vi "Initialize.vi"(7 "Simulate?":bool, 8 "error in (no error)":errorcluster, 10 "Port config":T1={"baud rate"=9600, "data bits"=8, "parity"=enum."None", "stop bits"=0}, 11 "VISA Refnum in":refnum<visa-resource-name>) -> (0 "error out":errorcluster, 2 "Connected?":bool, 3 "VISA Refnum out":refnum<visa-resource-name>)   [LabVIEW 2020, in "Monochromator.lvlib"]
uses:
  Monochromator.lvlib
  <vilib>/Instr/_visa.llb/VISA Flush IO Buffer Mask.ctl
  <vilib>/Instr/_visa.llb/VISA Configure Serial Port (Instr).vi
panel:
  out "return count write":u32
  out "return count read":u32
  out "Data read":string
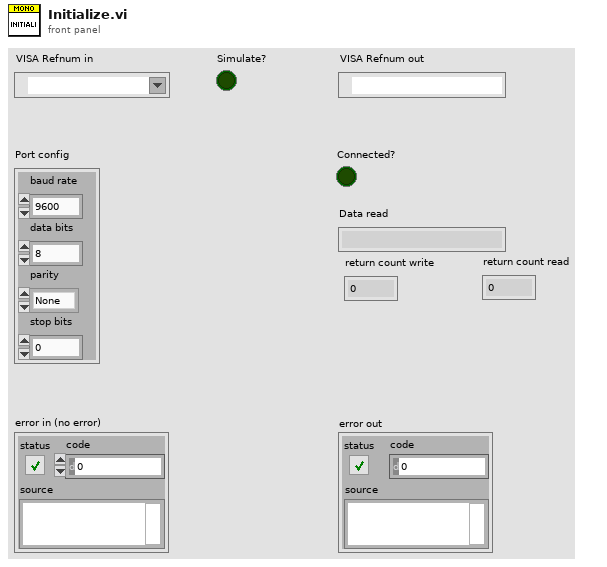
[diagram p1: front panel]
types:
  T1 = cluster{"baud rate":u32, "data bits":u16, "parity":enum16{"None", "Odd", "Even", "Mark", "Space"}, "stop bits":u16}
  T2 = typedef "VISA Flush IO Buffer Mask.ctl" = u16
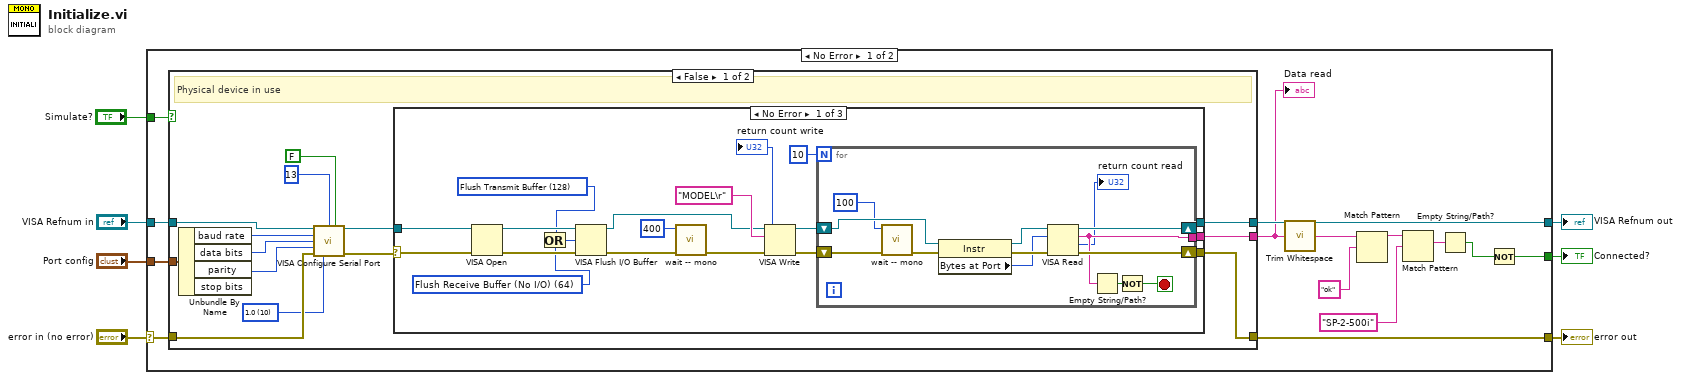
[diagram p0: block diagram]
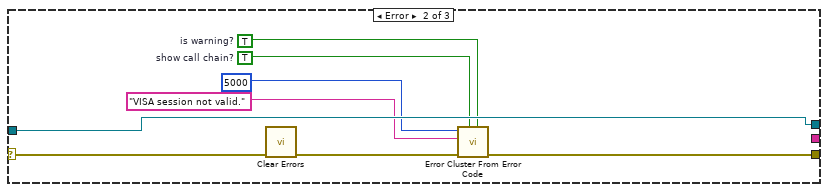
[diagram p2: hidden frame]
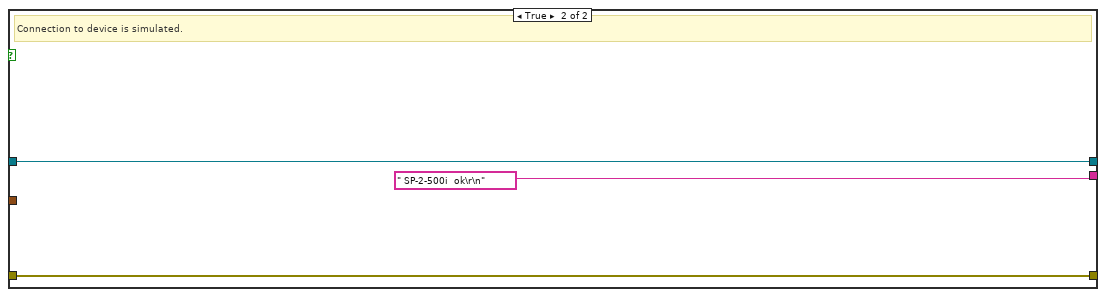
[diagram p4: hidden frame]
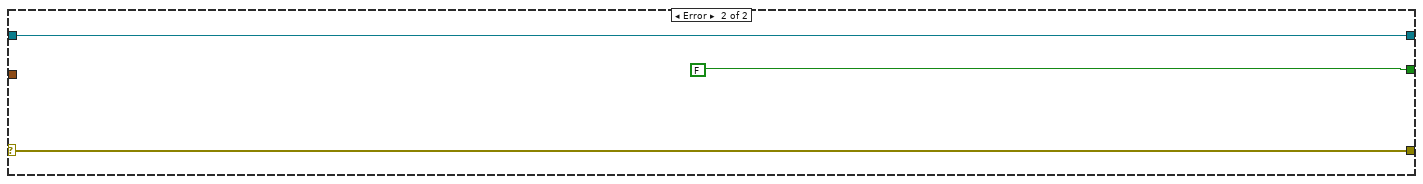
[diagram p5: hidden frame]
diagram:
  n1 = case shown="No Error" "error in (no error)" {
    selector: "error in (no error)" -> [w19 w82]
    tunnel: "Port config" -> [w21 _]
    tunnel: "VISA Refnum in" -> [w20 w83]
    tunnel: [w18 w82] -> w4
    tunnel: [w17 w83] -> w3
    tunnel: [w9 FALSE] -> w2
    tunnel: "Simulate?" -> [w8 _]
    frame No Error {
      n2 = case shown="False" w8 {
        tunnel: w21 -> [w35 _]
        tunnel: w20 -> [w34 w78]
        tunnel: w19 -> [w33 w79]
        tunnel: [w32 w79] -> w18
        tunnel: [w31 w78] -> w17
        tunnel: [w30 " SP-2-500i  ok\r\n" ("regular expression")] -> w15
        frame False {
          w25 = u16 10 items=["1.0"=10, "1.5"=15, "2.0"=20] ("stop bits (10: 1 bit)")
          # "Physical device in use"
          n3 = Unbundle By Name(w35) -> ("baud rate"=w27:u32, "data bits"=w28:u16, "parity"=w29:enum16{"None", "Odd", "Even", "Mark", "Space"})  [unwired: 1 out]
          n4 = call-poly "VISA Configure Serial Port"("VISA resource name"=w34, "termination char\n(0xA = '\\n' = LF)"=u8 13 ("termination char\n(0xA = '\\n' = LF)"), "Enable Termination\nChar (T)"=FALSE ("Enable Termination\nChar (T)"), "baud rate (9600)"=w27, "data bits (8)"=w28, "parity (0:none)"=w29, "error in (no error)"=w33, "stop bits (10: 1 bit)"=w25) -> ("VISA resource name out"=w24:refnum<visa-resource-name>, "error out"=w23:errorcluster)  [unwired: 6 in]
          n5 = case shown="No Error" w23 {
            selector: w23 -> [w50 w74 w76]
            tunnel: [w54 w72 w76] -> w32
            tunnel: [w53 w75 w77] -> w31
            tunnel: [w52 _ _] -> w30
            tunnel: w24 -> [w51 w75 w77]
            frame No Error {
              w38 = T2 64 items=["Flush Receive Buffer"=16, "Write Transmit Buffer to Device"=32, "Flush Receive Buffer (No I/O)"=64, "Flush Transmit Buffer"=128] ("Mask")
              w39 = T2 128 items=["Flush Receive Buffer"=16, "Write Transmit Buffer to Device"=32, "Flush Receive Buffer (No I/O)"=64, "Flush Transmit Buffer"=128] ("Mask")
              n6 = VISA Open(error in (no error)=w50, VISA resource name=w51) -> (VISA resource name=w41:refnum<visa-resource-name>, error out=w43:errorcluster)  [unwired: 3 in]
              n7 = Or(x=w39, y=w38) -> (x .or. y?=w37:T2)
              n8 = VISA Flush I/O Buffer(VISA resource name=w41, mask (16)=w37, error in (no error)=w43) -> (VISA resource name out=w40:refnum<visa-resource-name>, error out=w42:errorcluster)
              n9 = call "wait -- mono.vi"("error in (no error)"=w42, "milliseconds to wait"=u32 400) -> ("error out"=w46:errorcluster)  [unwired: 9 in]
              n10 = VISA Write(VISA resource name=w40, write buffer="MODEL\r", error in (no error)=w46) -> (VISA resource name out=w49:refnum<visa-resource-name>, return count=→"return count write":u32, error out=w48:errorcluster)
              n11 = for {
                N: 10 -> [_]
                tunnel: [w58] -> w52
                shift-right: [w66] -> w53
                shift-left: w49 -> [w64]
                shift-right: [w67] -> w54
                shift-left: w48 -> [w62]
                stop <- w56 stop-if-true
                n12 = call "wait -- mono.vi"("error in (no error)"=w62, "milliseconds to wait"=u32 100) -> ("error out"=w61:errorcluster)  [unwired: 9 in]
                n13 = property class="Instr"(reference=w64, error in=w61) -> (reference out=w63:refnum<visa-resource-name>, error out=w65:errorcluster, "Bytes at Port"=w59:u32)
                n14 = VISA Read(VISA resource name=w63, byte count=w59, error in (no error)=w65) -> (VISA resource name out=w66:refnum<visa-resource-name>, read buffer=w58:string, return count=→"return count read":u32, error out=w67:errorcluster)
                n15 = Empty String/Path?(string/path=w58) -> (empty?=w57:bool)
                n16 = Not(x=w57) -> (.not. x?=w56:bool)
              }
            }
            frame Error {
              w68 = TRUE  # show call chain?
              w69 = TRUE  # is warning?
              n17 = call <vilib>:"Clear Errors.vi"("error in (no error)"=w74) -> ("error out"=w73:errorcluster)  [unwired: 5 in, 1 out]
              n18 = call <vilib>:"Error Cluster From Error Code.vi"("is warning? (False)"=w69, "show call chain? (False)"=w68, "error in (no error)"=w73, "error message (\"\")"="VISA session not valid." ("error message (\"\")"), "error code (0)"=5000) -> ("error out"=w72:errorcluster)  [unwired: 4 in]
            }
            frame Default {
            }
          }
        }
        frame True {
          # "Connection to device is simulated."
        }
      }
      "Data read" <- w15
      n19 = call <vilib>:"Trim Whitespace.vi"("string"=w15) -> ("trimmed string"=w14:string)  [unwired: 1 in]
      n20 = Match Pattern(string=w14, regular expression="ok") -> (before substring=w13:string)  [unwired: 1 in, 3 out]
      n21 = Match Pattern(string=w13, regular expression="SP-2-500i" ("y")) -> (match substring=w11:string)  [unwired: 1 in, 3 out]
      n22 = Empty String/Path?(string/path=w11) -> (empty?=w10:bool)
      n23 = Not(x=w10) -> (.not. x?=w9:bool)
    }
    frame Error {
    }
  }
  "VISA Refnum out" <- w3
  "error out" <- w4
  "Connected?" <- w2
